vi "Add XY point to Graph.vi"(8 "error in (no error)":errorcluster, 9 "Y":dbl, 10 "X":dbl, 11 "Graph in":refnum<vi>) -> (0 "error out":errorcluster, 3 "Graph out":refnum<vi>)   [LabVIEW 2018]
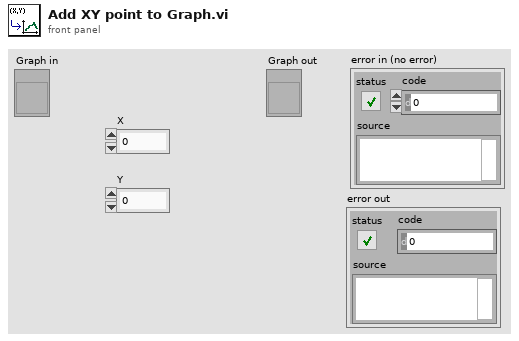
[diagram p1: front panel]
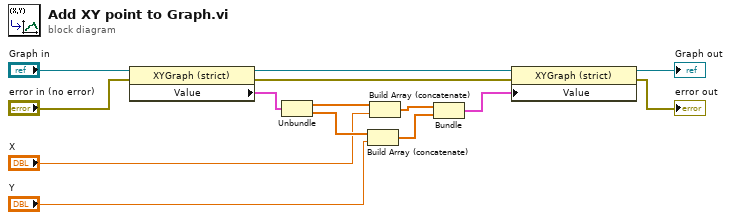
[diagram p0: block diagram]
diagram:
  n1 = property class="XYGraph (strict)"(reference="Graph in", error in="error in (no error)") -> (reference out=w7:refnum<vi>, error out=w5:errorcluster, "Value"=w12:cluster{dbl[], dbl[]})
  n2 = Unbundle(w12) -> (w11:dbl[], w10:dbl[])
  n3 = Build Array (concatenate)(w10, "Y") -> (w8:dbl[])
  n4 = Build Array (concatenate)(w11, "X") -> (w9:dbl[])
  n5 = Bundle(w9, w8) -> (w6:cluster{dbl[], dbl[]})  [unwired: 1 in]
  n6 = property class="XYGraph (strict)"(reference=w7, error in=w5, "Value"=w6) -> (reference out=→"Graph out":refnum<vi>, error out=→"error out":errorcluster)
